vi "Copy 7zSD.SFX.vi"(8 "error in (no error)":errorcluster, 11 "PostBuildSupport in":refnum<class "PostBuildSupport.lvclass">) -> (0 "error out":errorcluster, 3 "PostBuildSupport out":refnum<class "PostBuildSupport.lvclass">)   [LabVIEW 2016, in "PostBuildSupport.lvclass"]
uses:
  PostBuildSupport.lvclass
  PostBuildSupport.lvclass/PostBuildSupport.ctl
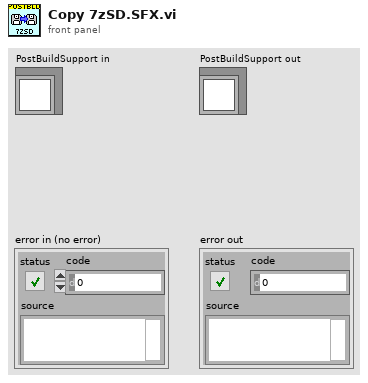
[diagram p1: front panel]
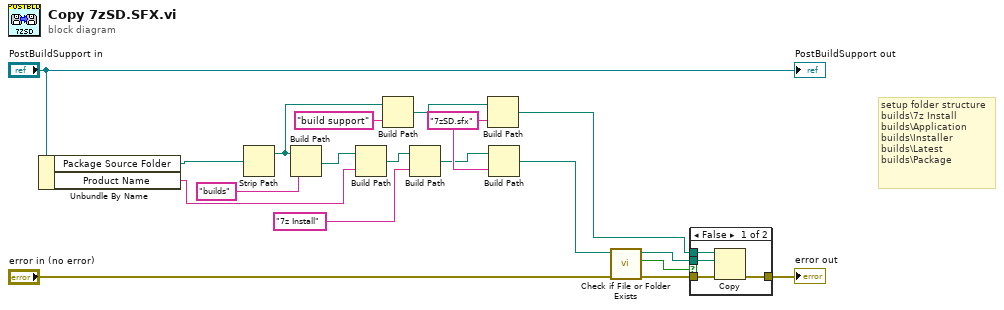
[diagram p0: block diagram]
diagram:
  w8 = "7zSD.sfx" ("name or relative path")
  # "setup folder structure\nbuilds\\7z Install\nbuilds\\Application\nbuilds\\Installer\nbuilds\\Latest\nbuilds\\Package"
  n1 = Unbundle By Name("PostBuildSupport in") -> ("Package Source Folder"=w16:path, "Product Name"=w15:string)
  n2 = Strip Path(path=w16) -> (stripped path=w9:path)  [unwired: 1 out]
  n3 = Build Path(base path=w9, name or relative path="builds") -> (appended path=w18:path)
  n4 = Build Path(base path=w18, name or relative path=w15) -> (appended path=w11:path)
  n5 = Build Path(base path=w9, name or relative path="build support") -> (appended path=w12:path)
  n6 = Build Path(base path=w11, name or relative path="7z Install") -> (appended path=w7:path)
  n7 = Build Path(base path=w12, name or relative path=w8) -> (appended path=w1:path)
  n8 = Build Path(base path=w7, name or relative path=w8) -> (appended path=w6:path)
  n9 = call <vilib>:"Check if File or Folder Exists.vi"("error in (no error)"="error in (no error)", "path"=w6) -> ("error out"=w3:errorcluster, "file or folder exists?"=w2:bool, "dup path"=w4:path)  [unwired: 7 in]
  n10 = case shown="False" w2 {
    tunnel: [w23 w24] -> w14
    tunnel: w1 -> [w22 _]
    tunnel: w4 -> [w21 _]
    tunnel: w3 -> [w20 w24]
    frame False {
      n11 = Copy(8:w20, 10:w21, 11:w22) -> (0:w23:errorcluster)  [unwired: 2 in, 2 out]
    }
    frame True {
    }
  }
  "error out" <- w14
  "PostBuildSupport out" <- "PostBuildSupport in"
